vi "Histeresis.vi"() -> ()   [LabVIEW 2020]
panel:
  out "Histeresis":bool
  out "x*y":dbl
  in  "stop":bool
  out "Rango":bool
  in  "min":dbl
  in  "max":dbl
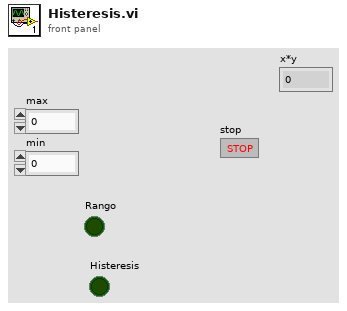
[diagram p1: front panel]
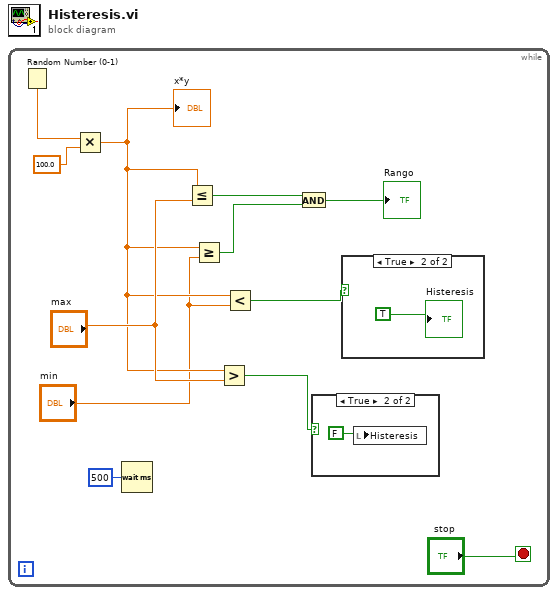
[diagram p0: block diagram]
diagram:
  n1 = while {
    stop <- "stop" stop-if-true
    n2 = Random Number (0-1)() -> (number: 0 to 1=w12:dbl)
    n3 = Multiply(x=w12, y=100.0) -> (x*y=w4:dbl)
    "x*y" <- w4
    n4 = Wait (ms)(milliseconds to wait=u32 500) -> ()  [unwired: 1 out]
    n5 = Less Or Equal?(x=w4, y="max") -> (x <= y?=w8:bool)
    n6 = Greater Or Equal?(x=w4, y="min") -> (x >= y?=w6:bool)
    n7 = Greater?(x=w4, y="max") -> (0:w1:bool)
    n8 = Less?(x=w4, y="min") -> (x < y?=w2:bool)
    n9 = And(x=w8, y=w6) -> (x .and. y?=→"Rango":bool)
    n10 = case shown="True" w1 {
      frame False {
      }
      frame True {
        n11 = local write "Histeresis"(FALSE) -> ()
      }
    }
    n12 = case shown="True" w2 {
      frame False {
      }
      frame True {
        "Histeresis" <- TRUE
      }
    }
  }
